vi "Actor Core.vi"(8 "error in":errorcluster, 11 "My Application":refnum<class "LogUI.lvclass">) -> (0 "error out":errorcluster, 3 "Actor out":refnum<class "Actor.lvclass">)   [LabVIEW 2014, in "EventsLogUI.lvlib" / "LogUI.lvclass"]
doc: "This is Actor Core.vi, the main message handling loop for Actors. An actor usually just sits in this loop and processes messages as they arrive. Any error returned by the message Do.vi call will stop the loop, with error code 43 as the canonical signal to stop with no error sent to caller. Descendants may override that in Handle Error.vi."
uses:
  LogUI.lvclass
  <vilib>/ActorFramework/Actor/Actor.lvclass
  JoyStick_lib/JoyStick/JoyStick.lvclass
  <vilib>/ActorFramework/Actor/Actor.lvclass/Actor.ctl
  <vilib>/ActorFramework/Message Enqueuer/Message Enqueuer.lvclass/Message Enqueuer.ctl
  LogUI.lvclass/LogUI.ctl
  <vilib>/ActorFramework/Message Enqueuer/Init from Existing Queue.vi
  <vilib>/ActorFramework/Message Enqueuer/Enqueue.vi
  <vilib>/ActorFramework/Message Priority Queue/Priority Enqueue.vi
  <vilib>/ActorFramework/Message Enqueuer/Message Enqueuer.lvclass
  UnitTest_lib/ChildActor/ChildActor.lvclass
  <vilib>/ActorFramework/Stop Msg/Stop Msg.lvclass
panel:
  in  "Message to State 3":bool
  in  "Message to State 2":bool
  in  "stop signal":bool
  out "Event Log":string
  in  "DNL_Stop":bool
  in  "Message to State":bool
  # "Change Debug Item when start?"
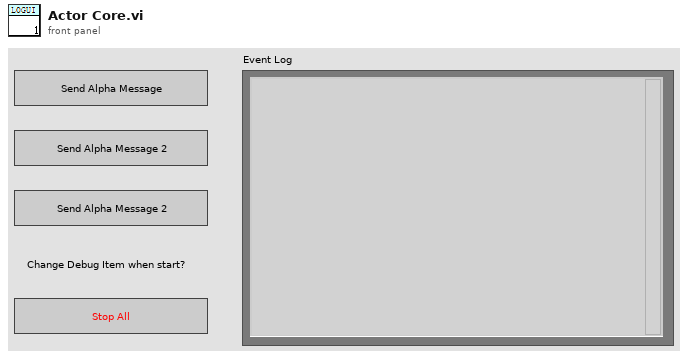
[diagram p1: front panel]
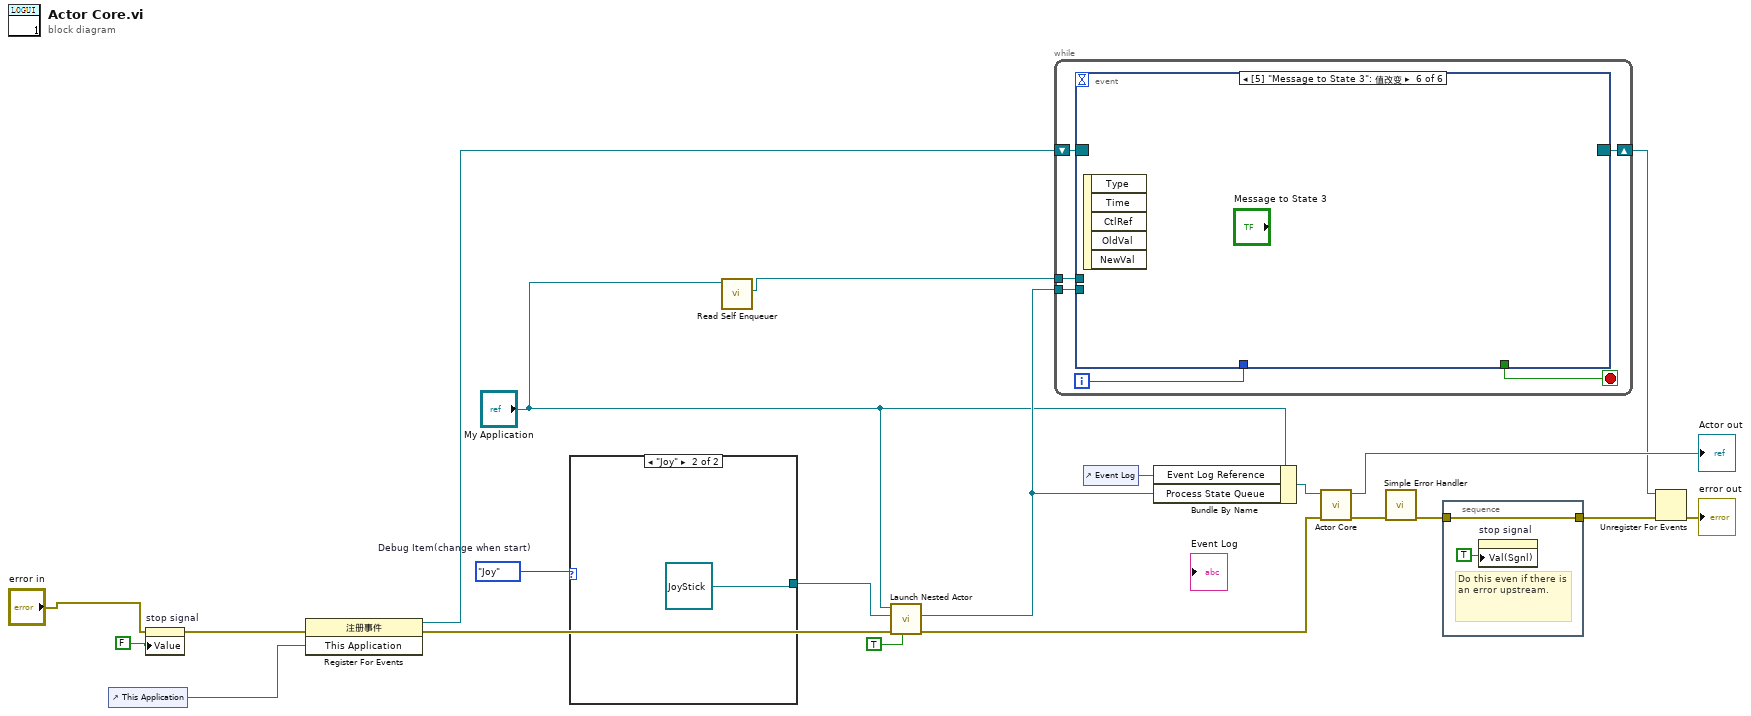
[diagram p0: block diagram]
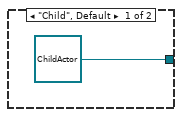
[diagram p2: hidden frame]
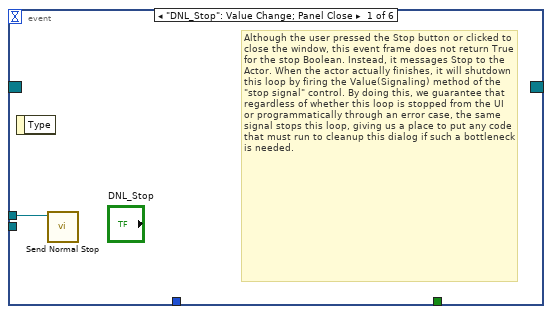
[diagram p3: hidden frame]
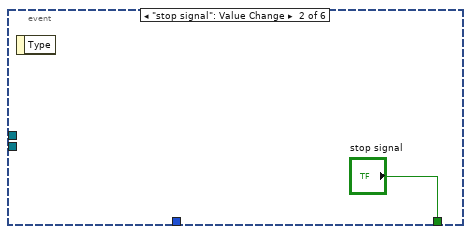
[diagram p4: hidden frame]
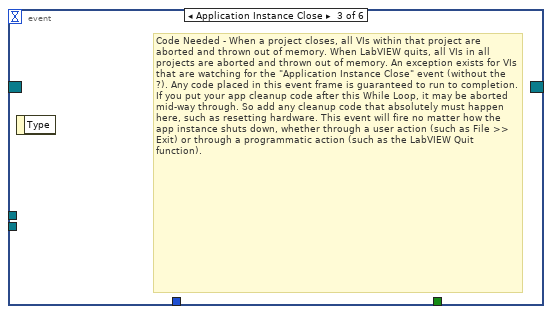
[diagram p5: hidden frame]
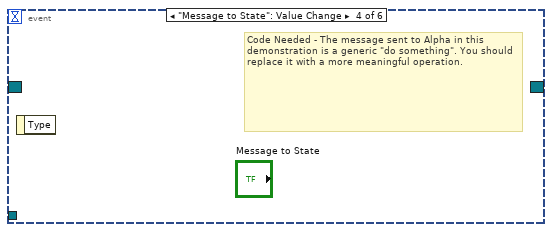
[diagram p6: hidden frame]
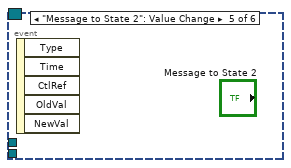
[diagram p7: hidden frame]
diagram:
  w1 = enum16{"Child", "Joy"}."Joy"  # Debug Item(change when start)
  n1 = control-ref of="This Application"() -> (w7:refnum<vi>)
  n2 = property on="stop signal" class="Bool (严格)"(error in="error in", "Value"=FALSE ("stop")) -> (error out=w9:errorcluster)  [unwired: 1 in, 1 out]
  n3 = register-events(error in=w9, w7) -> (reference out=w13:refnum<event-registration>, error out=w8:errorcluster)  [unwired: 1 in]
  n4 = case shown="\"Joy\"" w1 {
    tunnel: [refnum<class "ChildActor.lvclass"> refnum ("UnitTest.lvlib:ChildActor.lvclass") refnum<class "JoyStick.lvclass"> refnum ("JoyStick.lvlib:JoyStick.lvclass")] -> w3
    frame "Child", Default {
    }
    frame "Joy" {
    }
  }
  n5 = call <vilib>:"Read Self Enqueuer.vi"("Actor"="My Application") -> ("Self Enqueuer"=w17:refnum<class "Message Enqueuer.lvclass">)  [unwired: 10 in]
  n6 = call <vilib>:"Launch Nested Actor.vi"("Open Actor Core front panel? (F)"=TRUE, "error in (no error)"=w8, "Nested Actor"=w3, "Caller Actor in"="My Application") -> ("error out"=w20:errorcluster, "Nested Actor's Enqueuer"=w6:refnum<class "Message Enqueuer.lvclass">)  [unwired: 5 in, 1 out]
  n7 = while {
    tunnel: w17 -> [w29]
    tunnel: w6 -> [w28]
    shift-right: [w24] -> w12
    shift-left: w13 -> [w25]
    i -> [w26]
    stop <- w27 stop-if-true
    n8 = event shown="[5] \"Message to State 3\": 值改变" {
      selector: w25 -> [_ _ _ _ _ _]
      dyn-events: [_ _ _ _ _ _] -> w24
      timeout: _ -> [_ _ _ _ _ _]
      tunnel: w29 -> [w30 _ _ _ _ _]
      tunnel: w28 -> [_ _ _ _ _ _]
      tunnel: [_ "stop signal" _ _ _ _] -> w27
      tunnel: w26 -> [_ _ _ _ _ _]
      event "DNL_Stop": Value Change; Panel Close {
        # "Although the user pressed the Stop button or clicked to close the window, this event frame does not return True for the stop Boolean. Instead, it messages Stop to the Actor. When the actor actually finishes, it will shutdown this loop by firing the Value(Signaling) method of the \"stop signal\" control. By doing this, we guarantee that regardless of whether this loop is stopped from the UI or programmatically through an error case, the same signal stops this loop, giving us a place to put any code that must run to cleanup this dialog if such a bottleneck is needed."
        n9 = event-data() -> ()  [unwired: 1 in, 1 out]
        n10 = call <vilib>:"Send Normal Stop.vi"("Message Enqueuer"=w30) -> ()  [unwired: 10 in, 1 out]
      }
      event "stop signal": Value Change {
        n11 = event-data() -> ()  [unwired: 1 in, 1 out]
      }
      event Application Instance Close {
        # "Code Needed - When a project closes, all VIs within that project are aborted and thrown out of memory. When LabVIEW quits, all VIs in all projects are aborted and thrown out of memory. An exception exists for VIs that are watching for the \"Application Instance Close\" event (without the ?). Any code placed in this event frame is guaranteed to run to completion. If you put your app cleanup code after this While Loop, it may be aborted mid-way through. So add any cleanup code that absolutely must happen here, such as resetting hardware. This event will fire no matter how the app instance shuts down, whether through a user action (such as File >> Exit) or through a programmatic action (such as the LabVIEW Quit function)."
        n12 = event-data() -> ()  [unwired: 1 in, 1 out]
      }
      event "Message to State": Value Change {
        # "Code Needed - The message sent to Alpha in this demonstration is a generic \"do something\". You should replace it with a more meaningful operation."
        n13 = event-data() -> ()  [unwired: 1 in, 1 out]
      }
      event "Message to State 2": Value Change {
        n14 = event-data() -> ()  [unwired: 1 in, 5 out]
      }
      event "Message to State 3": Value Change {
        n15 = event-data() -> ()  [unwired: 1 in, 5 out]
      }
    }
  }
  n16 = control-ref of="Event Log"() -> (w18:refnum<vi>)
  n17 = Bundle By Name(cluster="My Application", "Event Log Reference"=w18, "Process State Queue"=w6) -> (w19:refnum<class "LogUI.lvclass">)
  n18 = call-parent "Actor Core.vi"("error in"=w20, "Actor in"=w19) -> ("error out"=w15:errorcluster, "Actor out"=→"Actor out":refnum<class "Actor.lvclass">)  [unwired: 8 in]
  n19 = call <vilib>:"Simple Error Handler.vi"("error in (no error)"=w15) -> ("error out"=w14:errorcluster)  [unwired: 4 in, 4 out]
  n20 = stacked-sequence {
    tunnel: [w32] -> w11
    tunnel: w14 -> [w32]
    frame #0 {
      # "Do this even if there is an error upstream."
      n21 = property on="stop signal" class="Bool (严格)"("Val(Sgnl)"=TRUE ("stop")) -> ()  [unwired: 2 in, 2 out]
    }
  }
  n22 = Unregister For Events(event registration refnum=w12, error in=w11) -> (error out=→"error out":errorcluster)
